vi "PXI6733 noise 測試.vi"() -> ()   [LabVIEW 2010]
panel:
  in  "stop (F)":bool
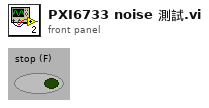
[diagram p1: front panel]
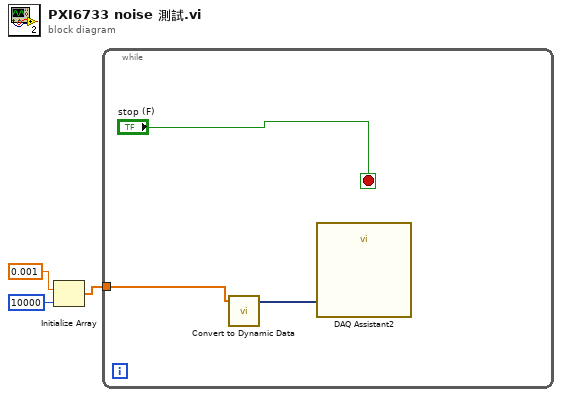
[diagram p0: block diagram]
diagram:
  n1 = Initialize Array(0.001 ("element"), 10000 ("dimension size")) -> (w3:dbl[])
  n2 = while {
    tunnel: w3 -> [w5]
    stop <- "stop (F)" stop-if-true
    n3 = call "Convert to Dynamic Data"("Array"=w5) -> ("Dynamic Data Type"=w6:dynamicdata)  [unwired: 3 in]
    n4 = call "DAQ Assistant2"("data"=w6) -> ()  [unwired: 16 in, 3 out]
  }
